vi "enable torque filtering.vi"(9 "Message handler data":T1, 11 "Data":variant) -> (0 "variant error":errorcluster)   [LabVIEW 2018]
doc: "The rateMultiplier option effectively changes the DAQ operating speed by skipping data transmits.\n\nThe base acquisition rate is 50kHz and setting the multiplier to 0 means every reading is trasmitted resulting in a rate of 50kHz. If the multiplier is set to 1 it returns every other reading resulting in a halving of the data rate (25kHZ)."
uses:
  Type Defs/Message loop data.ctl
  Type Defs/FPGA reference.ctl
  Type Defs/RT Status.ctl
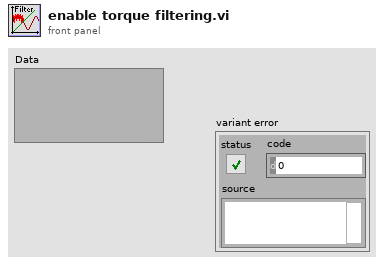
[diagram p1: front panel]
types:
  T1 = typedef "Message loop data.ctl" = cluster{"Parameters":cluster{"FPGA Ref":T2, "configID":u32, "activeChannels":cluster{"index":u16, "name":string}[]}, "Variables":cluster{"RT Status":T3, "watchdog":timestamp, "limitsEnabled":bool, "Interlocks":cluster{"gearboxOil":bool, "bearingOil":bool, "gearboxAir":bool}}}
  T2 = typedef "FPGA reference.ctl" = refnum<k20>
  T3 = typedef "RT Status.ctl" = cluster{"Comms loop":bool, "scheduler loop":bool, "data process loop":bool, "FIFO loop":bool, "Command Stream":bool, "Error Stream":bool, "FPGA FIFO":bool, "Data Stream":bool}
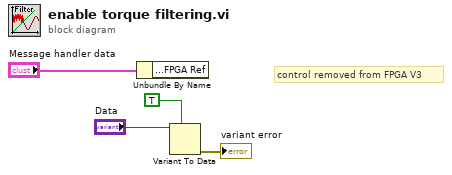
[diagram p0: block diagram]
diagram:
  # "control removed from FPGA V3"
  n1 = Unbundle By Name("Message handler data") -> ()  [unwired: 1 out]
  n2 = Variant To Data(type=TRUE, Variant="Data") -> (error out=→"variant error":errorcluster)  [unwired: 1 in, 1 out]
